vi "TdmsReadData.vi"() -> ()   [LabVIEW 2010]
panel:
  out "property value":i32
  out "data 2":dbl[](array[numeric])
  out "data":timestamp[](array[timestamp])
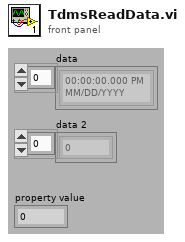
[diagram p1: front panel]
types:
  T1 = enum16{"open", "open or create", "create or replace", "create", "open (read-only)"}
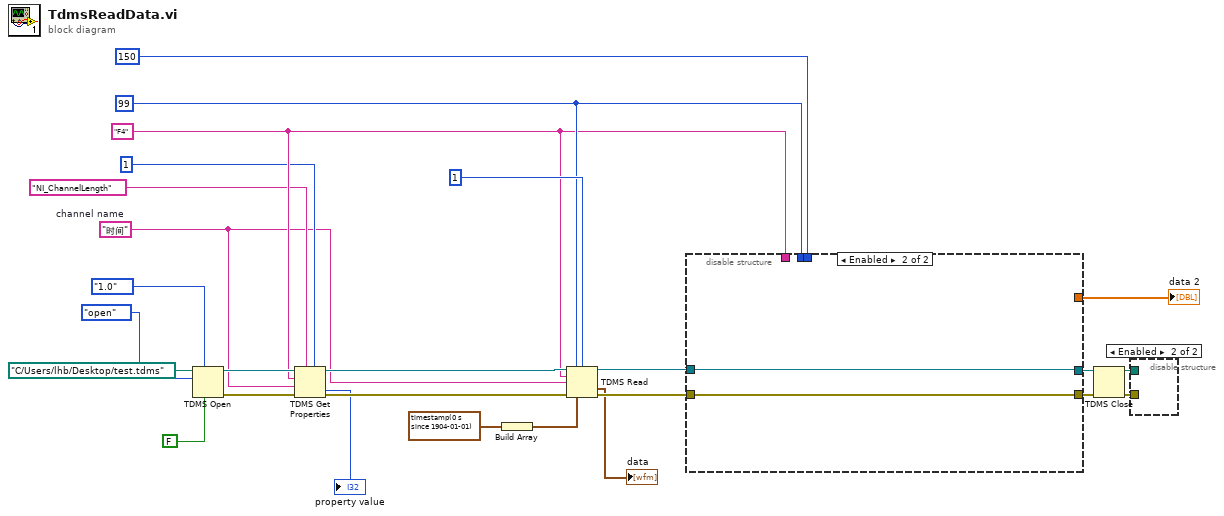
[diagram p0: block diagram]
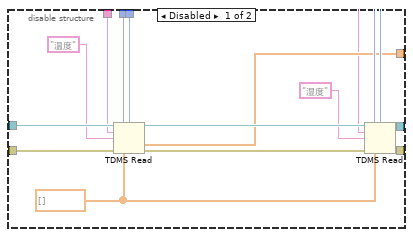
[diagram p2: hidden frame]
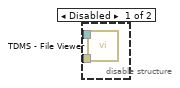
[diagram p3: hidden frame]
diagram:
  w2 = "时间"  # channel name
  w14 = i64 99 ("offset (0)")
  w6 = "F4" ("group name in")
  n1 = TDMS Open(6:FALSE ("disable buffering? (T)"), 7:enum16{"1.0", "2.0"}."1.0" ("file format version (2.0)"), 10:T1."open" ("operation (0:open)"), 11:path "C:/Users/lhb/Desktop/test.tdms" ("file path")) -> (0:w8:errorcluster, 3:w10:refnum<k34>)  [unwired: 2 in]
  n2 = TDMS Get Properties(5:1 ("index"), 7:"NI_ChannelLength" ("property name"), 8:w8, 9:w2, 10:w6, 11:w10) -> (0:w7:errorcluster, 3:w9:refnum<k34>, 4:→"property value":i32)  [unwired: 3 out]
  n3 = Build Array(timestamp(0 s since 1904-01-01) ("current time")) -> (w19:timestamp[])
  n4 = TDMS Read(0:w9, 1:w14, 2:i64 1 ("count (-1: all)"), 5:w6, 7:w2, 11:w7, 12:w19) -> (4:w17:refnum<k34>, 10:→"data":timestamp[], 15:w18:errorcluster)  [unwired: 3 out]
  n5 = disable-structure shown="Enabled" {
    disable-tunnel: w18 -> [w39 w40]
    disable-tunnel: w17 -> [w36 w41]
    disable-tunnel: [w35 w41] -> w16
    disable-tunnel: [w34 w40] -> w15
    disable-tunnel: w14 -> [w32 _]
    disable-tunnel: i64 150 ("count (-1: all)") -> [w31 _]
    disable-tunnel: [w30 _] -> w11
    disable-tunnel: w6 -> [w27 _]
    frame Disabled {
      w33 = dbl[] [] ("appended array")
      n6 = TDMS Read(0:w36, 1:w32, 2:w31, 5:w27, 7:"温度", 11:w39, 12:w33) -> (4:w38:refnum<k34>, 10:w30:dbl[], 15:w37:errorcluster)  [unwired: 3 out]
      n7 = TDMS Read(0:w38, 1:w32, 2:w31, 5:w27, 7:"湿度", 11:w37, 12:w33) -> (4:w35:refnum<k34>, 15:w34:errorcluster)  [unwired: 4 out]
    }
    frame Enabled {
    }
  }
  "data 2" <- w11
  n8 = TDMS Close(8:w15, 11:w16) -> (0:w21:errorcluster, 3:w22:path)
  n9 = disable-structure shown="Enabled" {
    disable-tunnel: w22 -> [w43 _]
    disable-tunnel: w21 -> [w42 _]
    frame Disabled {
      n10 = call <vilib>:"TDMS - File Viewer.vi"("error in (no error)"=w42, "file path"=w43) -> ()  [unwired: 6 out]
    }
    frame Enabled {
    }
  }
